vi "H5_CloseFile.vi"(8 "error in (no error)":errorcluster, 10 "HDF5 Dataset Ref":T1, 11 "HDF5 Ref":T1) -> (0 "error out":errorcluster)   [LabVIEW 2020]
uses:
  <vilib>/UPVI/lvhdf5/library.llb/HDF5 Ref.ctl
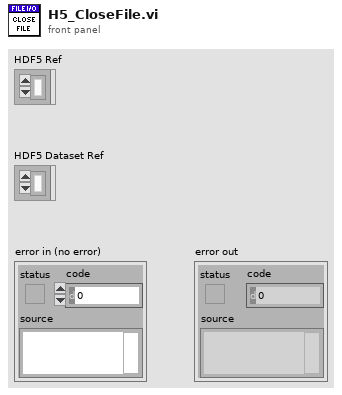
[diagram p1: front panel]
types:
  T1 = typedef "HDF5 Ref.ctl" = refnum<k1>
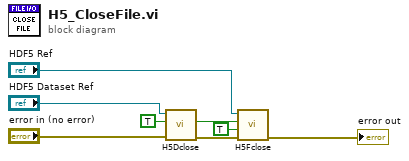
[diagram p0: block diagram]
diagram:
  n1 = call <vilib>:"H5Dclose.vi"("error in (no error)"="error in (no error)", "HDF5 Dataset Ref"="HDF5 Dataset Ref") -> ("error out"=w7:errorcluster)  [unwired: 7 in]
  n2 = call <vilib>:"H5Fclose.vi"("error in (no error)"=w7, "Force Close (F)"=TRUE, "Close All Open Objects (T)"=TRUE, "HDF5 Ref"="HDF5 Ref") -> ("error out"=→"error out":errorcluster)  [unwired: 5 in]
